vi "Get Controller Card Model.vi"(11 "controllerCardModel":string) -> (2 "function return":u32, 3 "controllerCardModel out":string)   [LabVIEW 2018, in "AndorSDK.lvlib"]
doc: "EXPNETTYPE unsigned int WINAPI GetControllerCardModel(char * controllerCardModel);"
uses:
  AndorSDK.lvlib
  ATMCD32D.dll
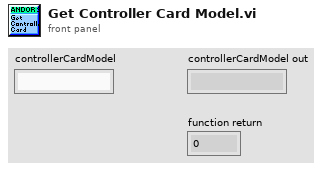
[diagram p1: front panel]
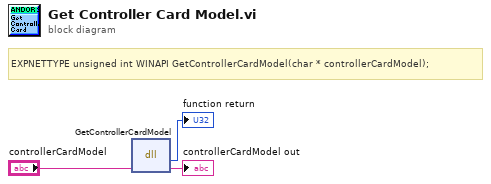
[diagram p0: block diagram]
diagram:
  # "EXPNETTYPE unsigned int WINAPI GetControllerCardModel(char * controllerCardModel);"
  n1 = dll-call lib="PTH2babs E\nPersönliches02 - Arbeit03-HiwijobsLabviewCodelibANDOR\tAndor SDK\nATMCD32D.*" fn="GetControllerCardModel"("controllerCardModel"="controllerCardModel") -> (→"function return":u32, "controllerCardModel"=→"controllerCardModel out":string)  [unwired: 3 in, 2 out]
